vi "MGCC_FntStaMach_gobal.vi"() -> ()   [LabVIEW 2016]
panel:
  out "f_MGCC_OnliTopolden_EnergizedMatrix":dbl[](array[numeric])
  in  "b_MGCC_fntStaMach_all_loop_stop":bool
  in  "b_MGCC_fntStaMach_communication_working":bool
  in  "b_MGCC_fntStaMach_ModelMgmt_done":bool
  in  "s_MGCC_FntStaMach_vis":string[](array[string])
  out "f_MGCC_FntStaMach_node":dbl[](array[numeric])
  out "f_MGCC_BKS_command":dbl[][](array[numeric])
  in  "s_MGCC_FntStaMach_State":string[](array[string])
  out "f_MGCC_OnliTopolden_node":dbl[][](array[numeric])
  in  "Enable_All":bool[][](array[boolean])
  in  "b_MGCC_fntStaMach_IsdCon_Enable":bool[](array[boolean])
  in  "b_MGCC_fntStaMach_Resync_Enable":bool[](array[boolean])
  in  "b_MGCC_fntStaMach_UnPlannedISD_Enable":bool[](array[boolean])
  in  "b_MGCC_fntStaMach_PlanISD_Enable":bool[](array[boolean])
  in  "b_MGCC_fntStaMach_DataLog_Enable":bool[](array[boolean])
  in  "b_MGCC_fntStaMach_PVFcst_Enable":bool[](array[boolean])
  in  "b_MGCC_fntStaMach_EnergyMgmt_Enable":bool[](array[boolean])
  in  "b_MGCC_fntStaMach_LoadFcst_Enable":bool[](array[boolean])
  in  "b_MGCC_fntStaMach_BlkStart_Enable":bool[](array[boolean])
  in  "b_MGCC_fntStaMach_PQBal_Enable":bool[](array[boolean])
  in  "b_MGCC_fntStaMach_State_Estimation_Enable":bool[](array[boolean])
  in  "Function enable by fault/abnormal":bool[][](array[boolean])
  in  "b_MGCC_EnergyMgmt_DB_Enable":bool[](array[boolean])
  in  "b_MGCC_EnergyMgmt_OPT_Enable":bool[](array[boolean])
  in  "b_MGCC_EnergyMgmt_ED_Enable":bool[](array[boolean])
  in  "b_MGCC_EnergyMgmt_UC_Enable":bool[](array[boolean])
  in  "b_MGCC_FntStaMach_State":bool[][](array[boolean])
  in  "Check Time":bool[](array[boolean])
  in  "ISD Success":bool[](array[boolean])
  in  "Unplanned BKS":bool[](array[boolean])
  in  "Pre_State":string[](array[string])
  in  "b_MGCC_BlkStart_Output_Success_Flag":bool[](array[boolean])
  in  "b_MGCC_OnliTopolden_Island_Status":bool[](array[boolean])
  in  "b_MGCC_FntStaMach_Island_Planned_cmd":bool[](array[boolean])
  in  "b_MGCC_FntStaMach_Recon_cmd":bool[](array[boolean])
  in  "b_MGCC_FntStaMach_BKS_cmd":bool[](array[boolean])
  in  "Unplanned ISD":bool[](array[boolean])
  in  "Abnormal State Flag":bool[](array[boolean])
  in  "Fault State Flag":bool[](array[boolean])
  in  "b_MGCC_FntStaMach_ReadyToRun":bool[](array[boolean])
  in  "b_MGCC_FntStaMach_Event_Manually_Control":bool
  in  "b_MGCC_FntStaMach_Reset":bool[](array[boolean])
  in  "b_MGCC_FntStaMach_IsdCon_enable":bool
  in  "b_MGCC_FntStaMach_Resync_Enable":bool
  in  "b_MGCC_FntStaMach_BlkStart_Enable":bool
  in  "b_MGCC_FntStaMach_UnplannedISD_enable":bool
  in  "b_MGCC_FntStaMach_PlanISD_enable":bool
  in  "b_MGCC_FntStaMach_DataLog_enable":bool
  in  "b_MGCC_FntStaMach_PVFcst_Enable":bool
  in  "b_MGCC_FntStaMach_EnergyMgmt_Enable":bool
  in  "b_MGCC_FntStaMach_LoadFcst_Enable":bool
  in  "b_MGCC_FntStaMach_PQBal_enable":bool
  in  "b_MGCC_FntStaMach_state_estimation_enable":bool
  in  "Enable":bool[](array[boolean])
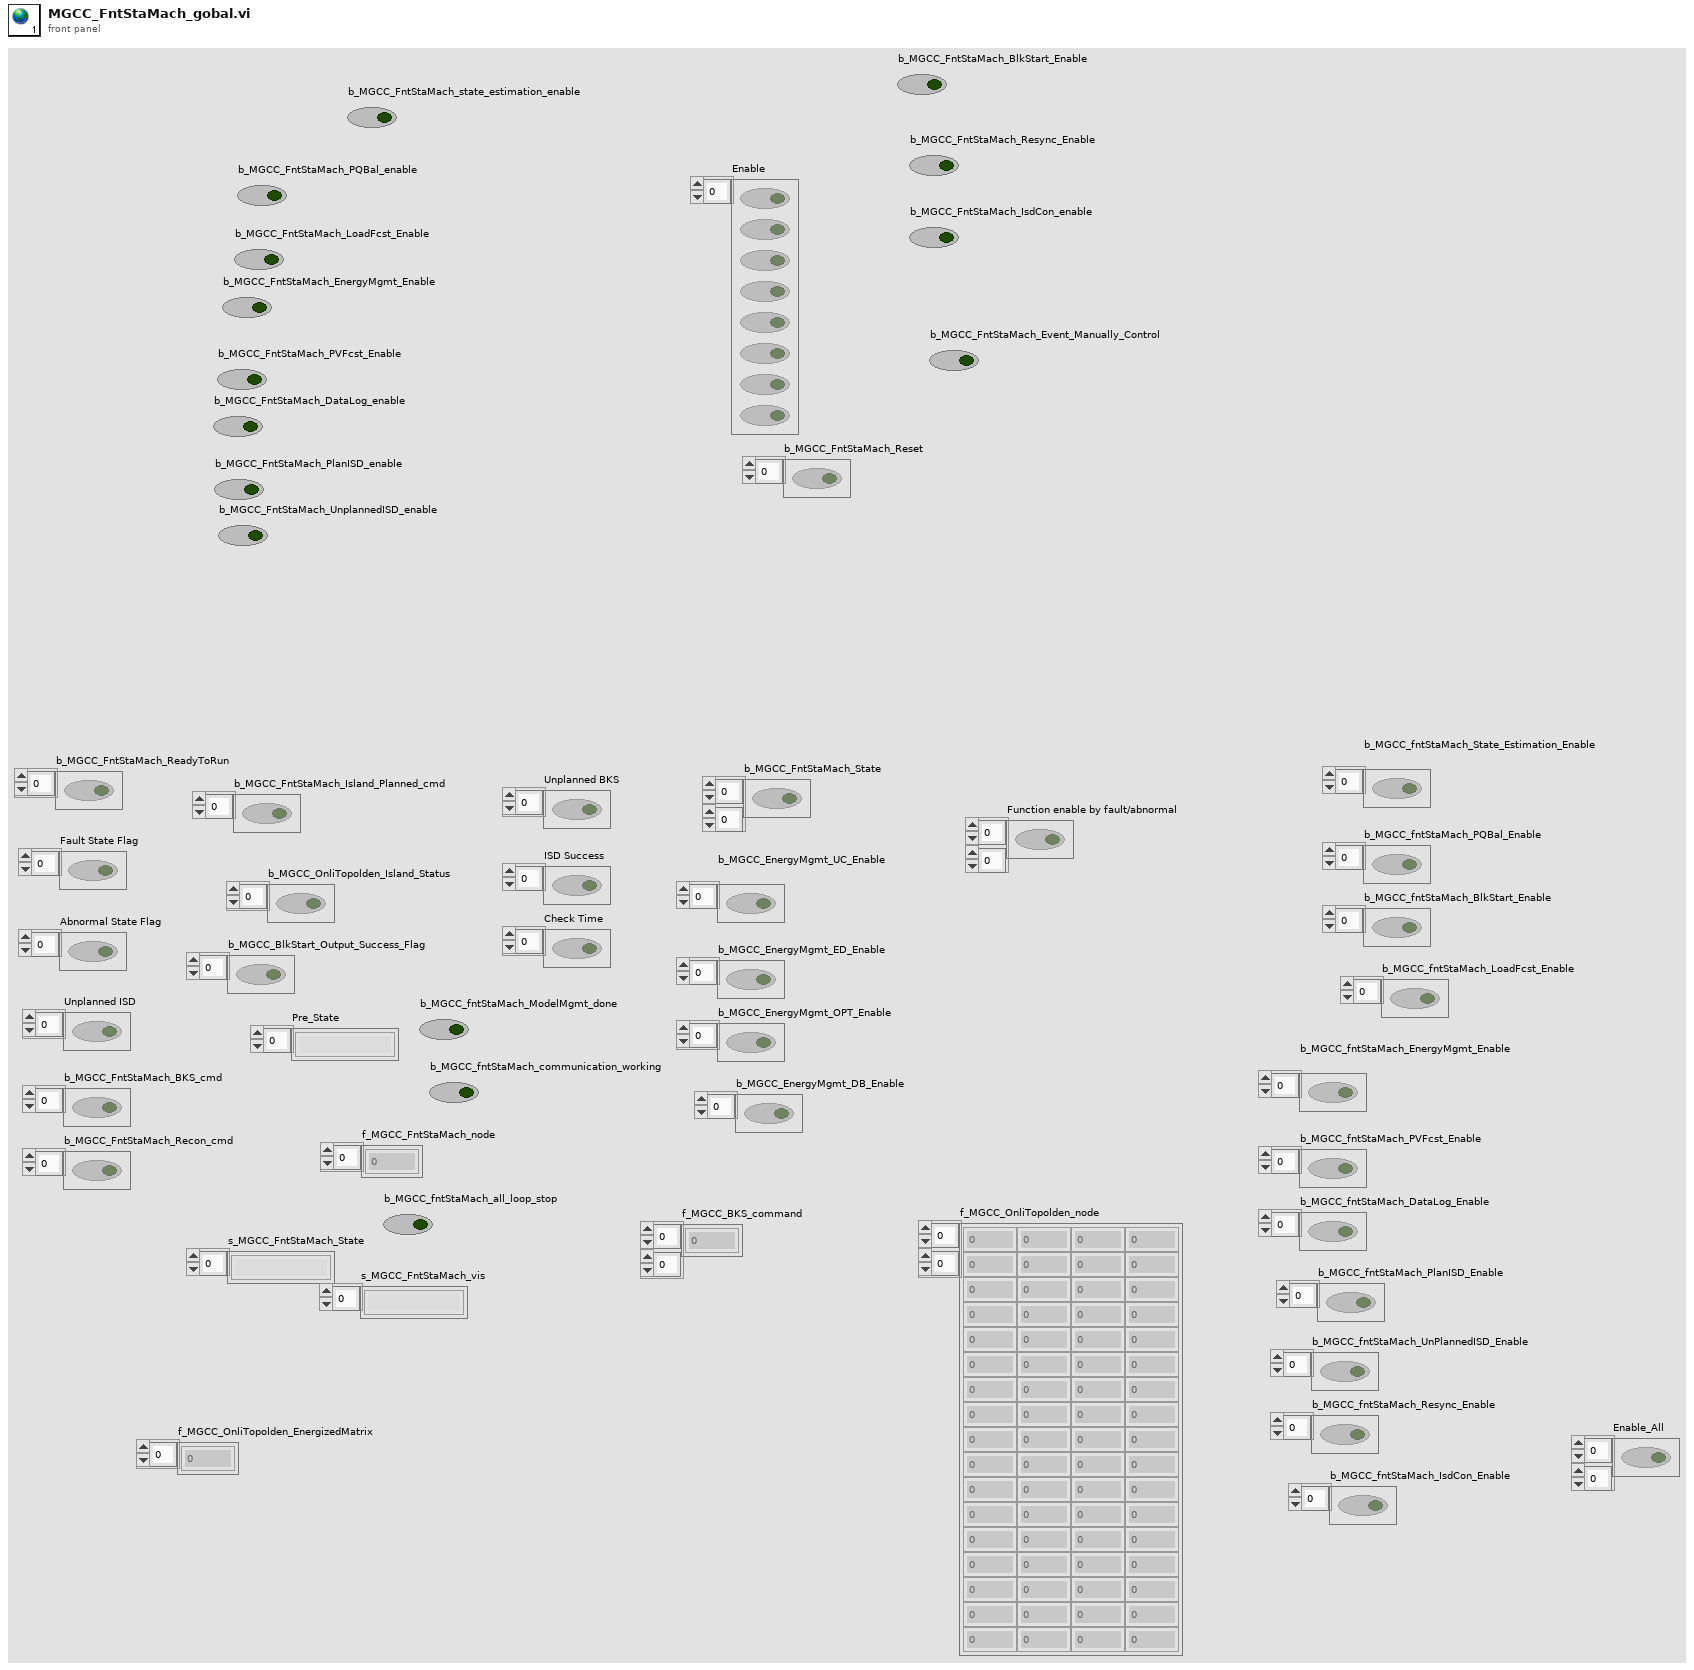
[diagram p1: front panel]
diagram:
